vi "prepare_plots.vi"(10 "data_array":dbl[][](array[numeric]), 11 "freq_array":dbl[](array[numeric])) -> (3 "plot_data":cluster{"freq_array":dbl[], "X2":dbl[]}[](array[cluster]))   [LabVIEW 2025]
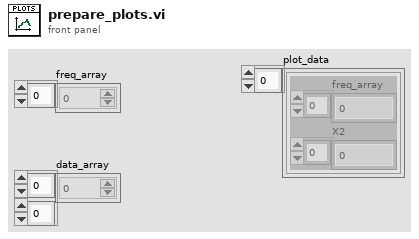
[diagram p1: front panel]
types:
  T1 = cluster{"vswr":dbl, "logmag":dbl, "phase":dbl, "R+jX_Norm":cluster{"R":dbl, "jX":dbl}, "R_Cap_Ind":cluster{"Rp":dbl, "Cp":dbl, "Lp":dbl, "Xp":dbl, "Cs":dbl, "Ls":dbl, "Z":dbl}, "R+jX_Scale":cluster{"R":dbl, "jX":dbl}, "power":dbl}
  T2 = cluster{"Rp":dbl, "Cp":dbl, "Lp":dbl, "Xp":dbl, "Cs":dbl, "Ls":dbl, "Z":dbl}
  T3 = cluster{"logmag":dbl, "phase":dbl, "R+jX_Norm":cluster{"R":dbl, "jX":dbl}, "R_Cap_Ind":cluster{"Rp":dbl, "Cp":dbl, "Lp":dbl, "Xp":dbl, "Cs":dbl, "Ls":dbl, "Z":dbl}, "group_delay":dbl, "trans_power":dbl}
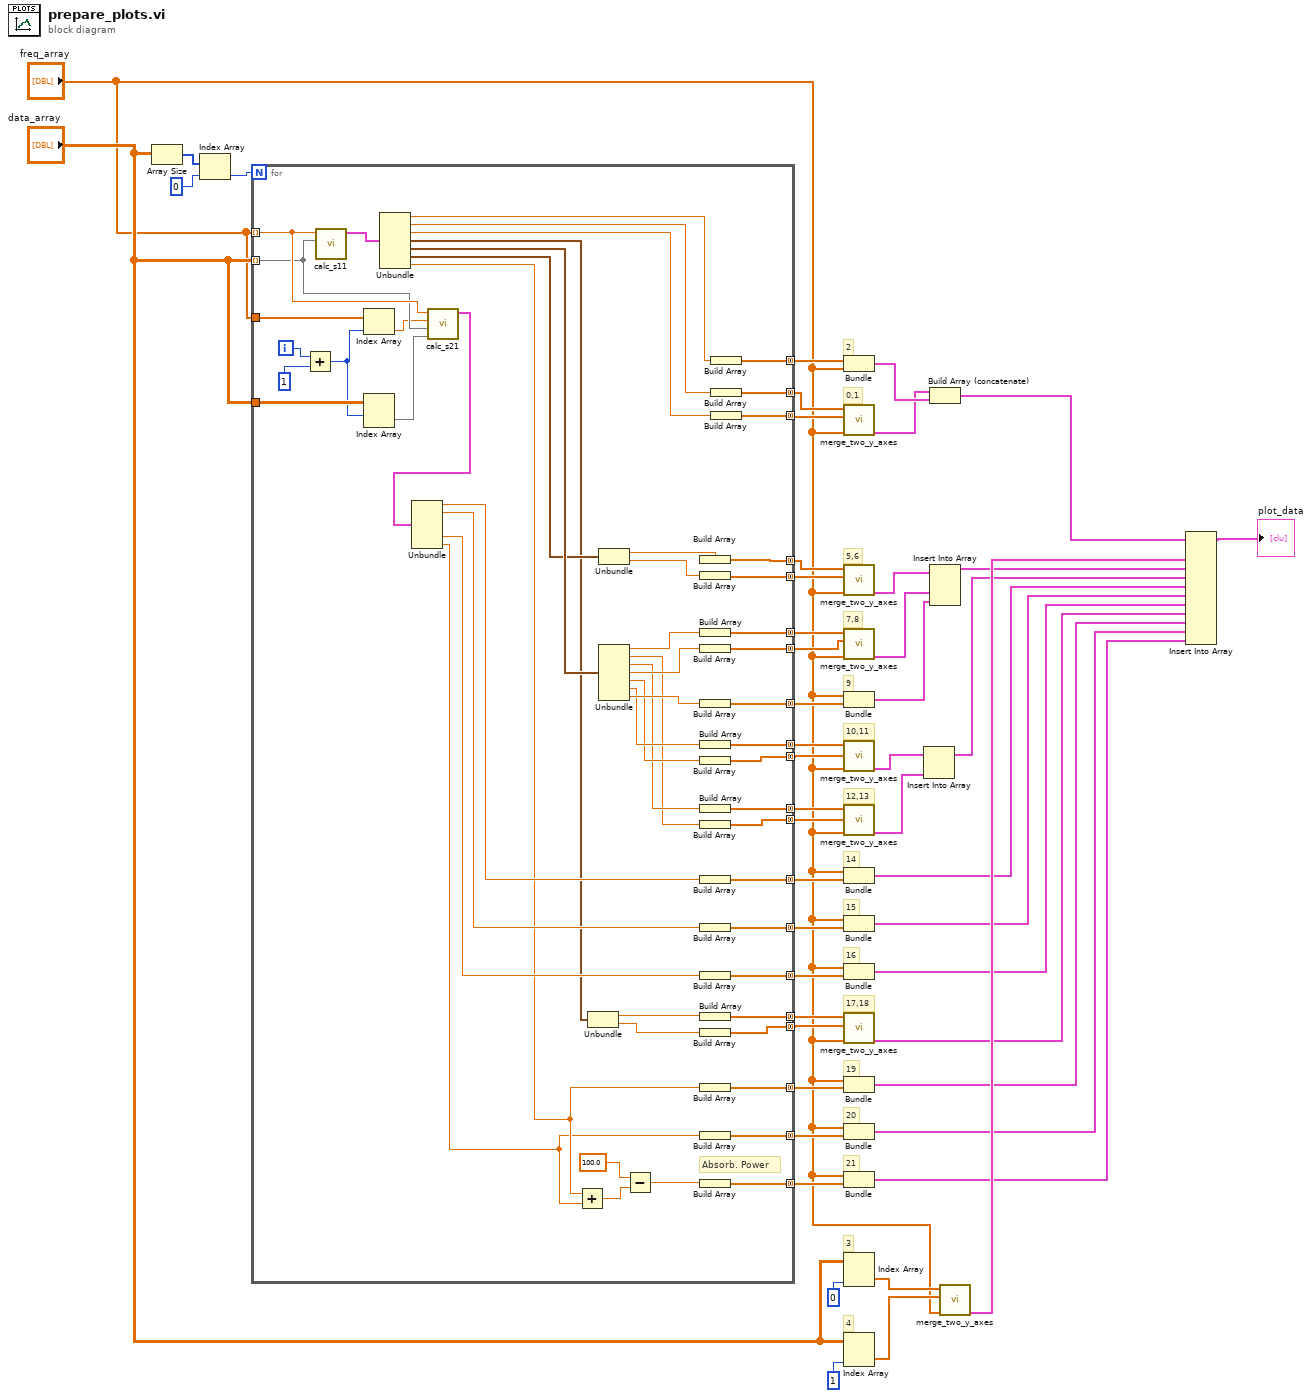
[diagram p0: block diagram]
diagram:
  # "21"
  # "20"
  # "4"
  # "3"
  # "19"
  # "17,18"
  # "16"
  # "15"
  # "14"
  # "12,13"
  # "10,11"
  # "9"
  # "7,8"
  # "5,6"
  # "0,1"
  # "2"
  n1 = Array Size(array="data_array") -> (size(s)=w44:i32[])
  n2 = Index Array(array=w44, index=0) -> (element=w46:i32)
  n3 = for {
    N: w46 -> [_]
    tunnel: "data_array" -> [w77] mode=indexing
    tunnel: "freq_array" -> [w78] mode=indexing
    tunnel: [w94] -> w39 mode=concatenating
    tunnel: [w95] -> w38 mode=concatenating
    tunnel: [w91] -> w36 mode=concatenating
    tunnel: [w89] -> w33 mode=concatenating
    tunnel: [w88] -> w32 mode=concatenating
    tunnel: [w87] -> w31 mode=concatenating
    tunnel: [w86] -> w30 mode=concatenating
    tunnel: [w103] -> w29 mode=concatenating
    tunnel: [w102] -> w28 mode=concatenating
    tunnel: [w101] -> w27 mode=concatenating
    tunnel: [w98] -> w25 mode=concatenating
    tunnel: [w97] -> w26 mode=concatenating
    tunnel: "freq_array" -> [w81]
    tunnel: "data_array" -> [w75]
    tunnel: [w69] -> w18 mode=concatenating
    tunnel: [w68] -> w16 mode=concatenating
    tunnel: [w66] -> w14 mode=concatenating
    tunnel: [w61] -> w11 mode=concatenating
    tunnel: [w60] -> w10 mode=concatenating
    tunnel: [w56] -> w7 mode=concatenating
    tunnel: [w55] -> w5 mode=concatenating
    tunnel: [w49] -> w3 mode=concatenating
    i -> [w80]
    # "Absorb. Power"
    n4 = Add(x=w80, y=1) -> (x+y=w74:i32)
    n5 = call "calc_s11.vi"("complex value"=w77, "frequency"=w78) -> ("s11_data"=w104:T1)  [unwired: 9 in]
    n6 = Index Array(array=w81, index=w74) -> (element=w76:dbl)
    n7 = Index Array(array=w75, index (row)=w74) -> (element=w73:dbl[])  [unwired: 1 in]
    n8 = Unbundle(w104) -> ("vswr"=w71:dbl, "logmag"=w100:dbl, "phase"=w99:dbl, "R+jX_Norm"=w57:cluster{"R":dbl, "jX":dbl}, "R_Cap_Ind"=w96:T2, "R+jX_Scale"=w62:cluster{"R":dbl, "jX":dbl}, "power"=w51:dbl)
    n9 = call "calc_s21.vi"("complex value+1"=w73, "complex value"=w77, "frequency+1"=w76, "frequency"=w78) -> ("s21_data"=w72:T3)  [unwired: 7 in]
    n10 = Unbundle(w72) -> ("logmag"=w70:dbl, "phase"=w65:dbl, "group_delay"=w67:dbl, "trans_power"=w50:dbl)  [unwired: 2 out]
    n11 = Add(x=w51, y=w50) -> (x+y=w53:dbl)
    n12 = Unbundle(w57) -> ("R"=w59:dbl, "jX"=w58:dbl)
    n13 = Unbundle(w62) -> ("R"=w64:dbl, "jX"=w63:dbl)
    n14 = Unbundle(w96) -> ("Rp"=w93:dbl, "Cp"=w82:dbl, "Lp"=w83:dbl, "Xp"=w92:dbl, "Cs"=w84:dbl, "Ls"=w85:dbl, "Z"=w90:dbl)
    n15 = Subtract(x=100.0, y=w53) -> (x-y=w52:dbl)
    n16 = Build Array(w64) -> (w98:dbl[])
    n17 = Build Array(w63) -> (w97:dbl[])
    n18 = Build Array(w93) -> (w94:dbl[])
    n19 = Build Array(w92) -> (w95:dbl[])
    n20 = Build Array(w90) -> (w91:dbl[])
    n21 = Build Array(w85) -> (w89:dbl[])
    n22 = Build Array(w84) -> (w88:dbl[])
    n23 = Build Array(w83) -> (w87:dbl[])
    n24 = Build Array(w82) -> (w86:dbl[])
    n25 = Build Array(w70) -> (w69:dbl[])
    n26 = Build Array(w65) -> (w66:dbl[])
    n27 = Build Array(w67) -> (w68:dbl[])
    n28 = Build Array(w59) -> (w61:dbl[])
    n29 = Build Array(w58) -> (w60:dbl[])
    n30 = Build Array(w51) -> (w56:dbl[])
    n31 = Build Array(w50) -> (w55:dbl[])
    n32 = Build Array(w52) -> (w49:dbl[])
    n33 = Build Array(w71) -> (w103:dbl[])
    n34 = Build Array(w100) -> (w102:dbl[])
    n35 = Build Array(w99) -> (w101:dbl[])
  }
  n36 = Bundle("freq_array"="freq_array", w29) -> (w23:cluster{"freq_array":dbl[], dbl[]})  [unwired: 1 in]
  n37 = call "merge_two_y_axes.vi"("X"="freq_array", "Y2"=w27, "Y1"=w28) -> ("graph_data"=w22:cluster{"Y":dbl[], "X2":dbl[]}[])  [unwired: 8 in]
  n38 = call "merge_two_y_axes.vi"("X"="freq_array", "Y2"=w26, "Y1"=w25) -> ("graph_data"=w41:cluster{"Y":dbl[], "X2":dbl[]}[])  [unwired: 8 in]
  n39 = call "merge_two_y_axes.vi"("X"="freq_array", "Y2"=w38, "Y1"=w39) -> ("graph_data"=w40:cluster{"Y":dbl[], "X2":dbl[]}[])  [unwired: 8 in]
  n40 = Bundle("freq_array"="freq_array", w36) -> (w37:cluster{"freq_array":dbl[], dbl[]})  [unwired: 1 in]
  n41 = call "merge_two_y_axes.vi"("X"="freq_array", "Y2"=w32, "Y1"=w33) -> ("graph_data"=w35:cluster{"Y":dbl[], "X2":dbl[]}[])  [unwired: 8 in]
  n42 = call "merge_two_y_axes.vi"("X"="freq_array", "Y2"=w30, "Y1"=w31) -> ("graph_data"=w34:cluster{"Y":dbl[], "X2":dbl[]}[])  [unwired: 8 in]
  n43 = Bundle("freq_array"="freq_array", w18) -> (w17:cluster{"freq_array":dbl[], dbl[]})  [unwired: 1 in]
  n44 = Bundle("freq_array"="freq_array", w14) -> (w13:cluster{"freq_array":dbl[], dbl[]})  [unwired: 1 in]
  n45 = Bundle("freq_array"="freq_array", w16) -> (w15:cluster{"freq_array":dbl[], dbl[]})  [unwired: 1 in]
  n46 = call "merge_two_y_axes.vi"("X"="freq_array", "Y2"=w10, "Y1"=w11) -> ("graph_data"=w9:cluster{"Y":dbl[], "X2":dbl[]}[])  [unwired: 8 in]
  n47 = Bundle("freq_array"="freq_array", w7) -> (w6:cluster{"freq_array":dbl[], dbl[]})  [unwired: 1 in]
  n48 = Bundle("freq_array"="freq_array", w5) -> (w4:cluster{"freq_array":dbl[], dbl[]})  [unwired: 1 in]
  n49 = Bundle("freq_array"="freq_array", w3) -> (w2:cluster{"freq_array":dbl[], dbl[]})  [unwired: 1 in]
  n50 = Index Array(array="data_array", index (col)=0) -> (element=w43:dbl[])  [unwired: 1 in]
  n51 = Index Array(array="data_array", index (col)=1) -> (element=w42:dbl[])  [unwired: 1 in]
  n52 = Insert Into Array(array=w35, new element=w34) -> (w19:cluster{"Y":dbl[], "X2":dbl[]}[])  [unwired: 1 in]
  n53 = Build Array (concatenate)(w22, w23) -> (w21:cluster{"freq_array":dbl[], "X2":dbl[]}[])
  n54 = Insert Into Array(array=w41, new element #1=w40, new element #2=w37) -> (w12:cluster{"Y":dbl[], "X2":dbl[]}[])  [unwired: 1 in]
  n55 = call "merge_two_y_axes.vi"("X"="freq_array", "Y2"=w42, "Y1"=w43) -> ("graph_data"=w20:cluster{"Y":dbl[], "X2":dbl[]}[])  [unwired: 8 in]
  n56 = Insert Into Array(array=w21, new element #1=w20, new element #2=w12, new element #3=w19, new element #4=w17, new element #5=w13, new element #6=w15, new element #7=w9, new element #8=w6, new element #9=w4, new element #10=w2) -> (→"plot_data":cluster{"freq_array":dbl[], "X2":dbl[]}[])  [unwired: 1 in]
